vi "Engine Out - Faults - Intake Air Temp.vi"(11 "Intake Air Temperature [C]":sgl) -> ()   [LabVIEW 2015, in "ECS-RT.lvlib"]
uses:
  ECS-RT.lvlib
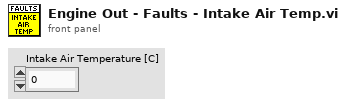
[diagram p1: front panel]
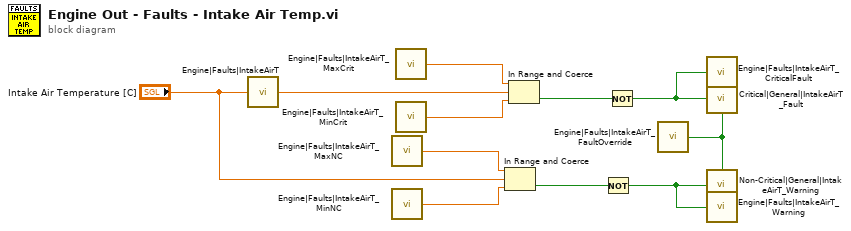
[diagram p0: block diagram]
diagram:
  n1 = call "Engine|Faults|IntakeAirT"("Value"="Intake Air Temperature [C]") -> ()
  n2 = call "Engine|Faults|IntakeAirT_MaxNC"() -> ("Value"=w7:sgl)
  n3 = call "Engine|Faults|IntakeAirT_MinNC"() -> ("Value"=w8:sgl)
  n4 = call "Engine|Faults|IntakeAirT_MaxCrit"() -> ("Value"=w3:sgl)
  n5 = call "Engine|Faults|IntakeAirT_MinCrit"() -> ("Value"=w4:sgl)
  n6 = In Range and Coerce(upper limit=w7, x="Intake Air Temperature [C]", lower limit=w8) -> (In Range?=w9:bool)  [unwired: 1 out]
  n7 = In Range and Coerce(upper limit=w3, x="Intake Air Temperature [C]", lower limit=w4) -> (In Range?=w5:bool)  [unwired: 1 out]
  n8 = Not(x=w9) -> (.not. x?=w10:bool)
  n9 = Not(x=w5) -> (.not. x?=w6:bool)
  n10 = call "Engine|Faults|IntakeAirT_FaultOverride"() -> ("Value"=w1:bool)
  n11 = call "Engine|Faults|IntakeAirT_CriticalFault"("Value"=w6) -> ()
  n12 = call "Critical|General|IntakeAirT_Fault"("Fault"=w6, "Override (F)"=w1) -> ()  [unwired: 1 in]
  n13 = call "Non-Critical|General|IntakeAirT_Warning"("Fault"=w10, "Override (F)"=w1) -> ()  [unwired: 1 in]
  n14 = call "Engine|Faults|IntakeAirT_Warning"("Value"=w10) -> ()
